vi "Compile Analog Replay Channels.vi"(5 "DAC bipolar range":dbl, 7 "Custom device ref":T1 format="%.0x", 8 "error in (no error)":errorcluster, 10 "1.0.0 Analog Replay in":T2, 11 "Item Ref in":T1 format="%.0x") -> (0 "error out":errorcluster, 2 "1.0.0 Analog Replay out":T2)   [LabVIEW 2013, in "Engine Simulation Toolkit System Explorer.lvlib"]
uses:
  Engine Simulation Toolkit System Explorer.lvlib
  Shared/1.0 Analog Replay Engine Data.ctl
  Shared/1.0 Analog Replay FIFO Idxs.ctl
  <vilib>/NI Veristand/Custom Device API/Custom Device Item Ref.ctl
  Shared/Constants and GUIDs.vi
  Shared/Properties.vi
  <vilib>/NI Veristand/Custom Device API/Get Item Property (Boolean).vi
  Shared/Engine Simulation Toolkit Shared.lvlib
  <vilib>/NI Veristand/Custom Device API/Custom Device API.lvlib
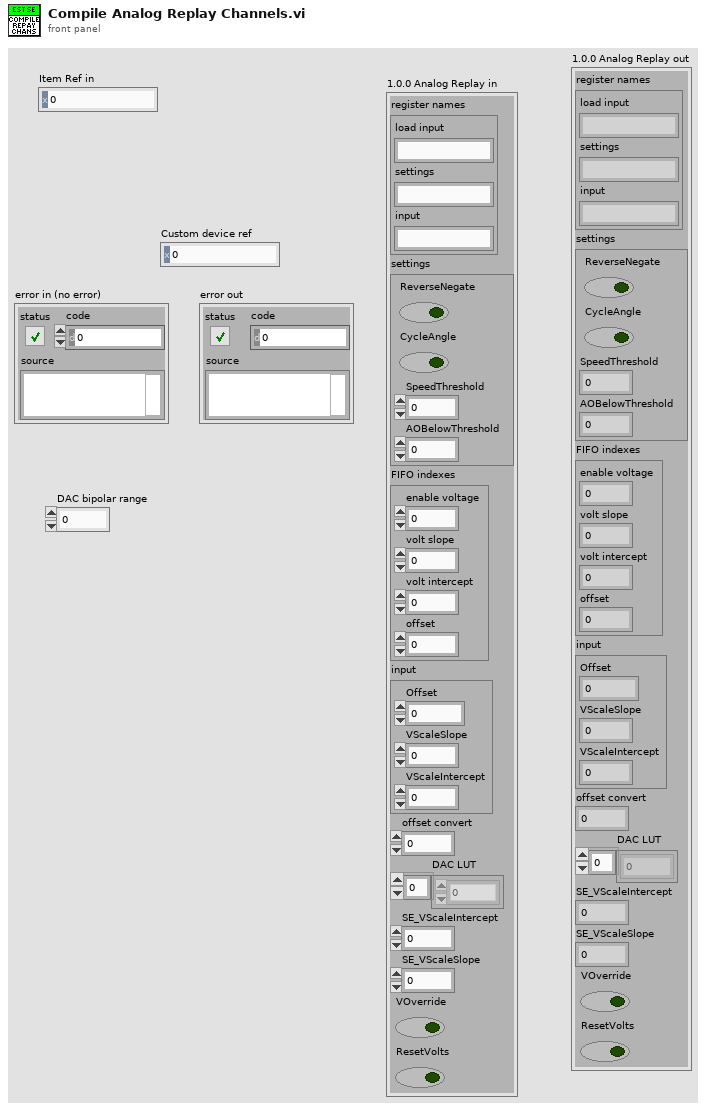
[diagram p1: front panel]
types:
  T1 = typedef "Custom Device API.lvlib/Custom Device Item Ref.ctl" = u64
  T2 = typedef "Engine Simulation Toolkit Shared.lvlib/1.0 Analog Replay Engine Data.ctl" = cluster{"register names":cluster{"load input":string, "settings":string, "input":string}, "settings":cluster{"ReverseNegate":bool, "CycleAngle":bool, "SpeedThreshold":fxp<+/-,23,2>, "AOBelowThreshold":i16}, "FIFO indexes":T3, "input":cluster{"Offset":i16, "VScaleSlope":fxp<+,18,6>, "VScaleIntercept":fxp<+/-,18,3>}, "offset convert":dbl, "DAC LUT":i16[], "SE_VScaleIntercept":fxp<+/-,18,3>, "SE_VScaleSlope":fxp<+,18,6>, "VOverride":bool, "ResetVolts":bool}
  T3 = typedef "Engine Simulation Toolkit Shared.lvlib/1.0 Analog Replay FIFO Idxs.ctl" = cluster{"enable voltage":i32, "volt slope":i32, "volt intercept":i32, "offset":i32}
  T4 = typedef "Engine Simulation Toolkit Shared.lvlib/Channel.ctl" = cluster{"Name":string, "Units":string, "Default":dbl, "Description":string}
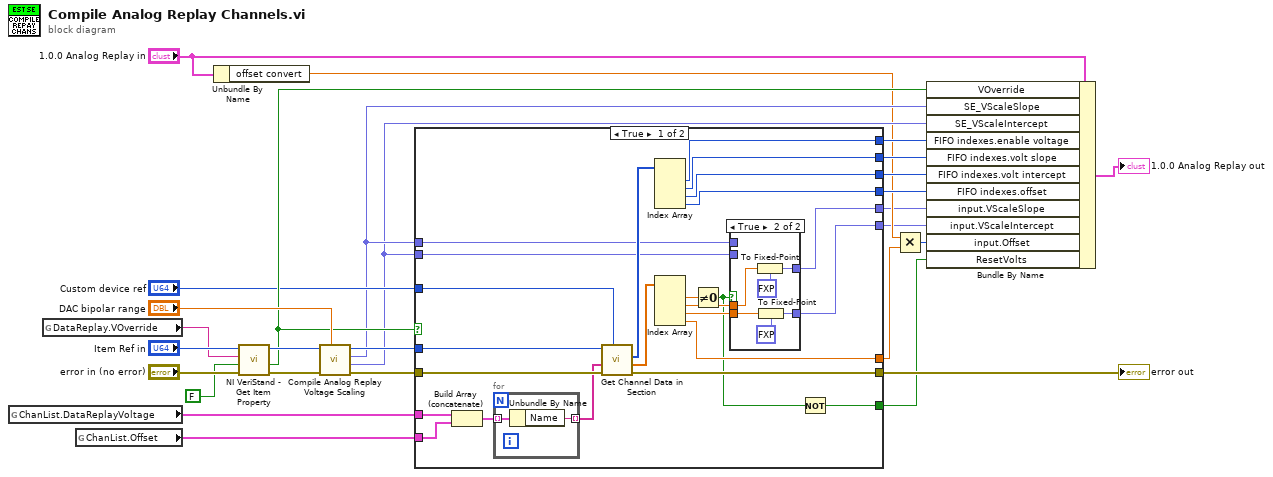
[diagram p0: block diagram]
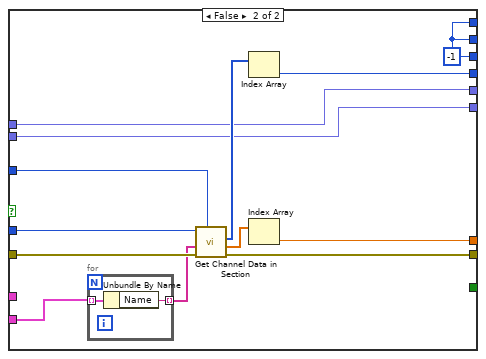
[diagram p3: hidden frame]
diagram:
  n1 = global read "Constants and GUIDs.vi" "ChanList.DataReplayVoltage"() -> (w20:T4[])
  n2 = global read "Properties.vi" "DataReplay.VOverride"() -> (w26:string)
  n3 = global read "Constants and GUIDs.vi" "ChanList.Offset"() -> (w19:T4[])
  n4 = Unbundle By Name("1.0.0 Analog Replay in") -> ("offset convert"=w5:dbl)
  n5 = call-poly <vilib>:"NI VeriStand - Get Item Property.vi"("error in (no error)"="error in (no error)", "Default Value"=FALSE, "Property Name"=w26, "Item Ref in"="Item Ref in") -> ("error out"=w23:errorcluster, "Value"=w21:bool, "Item Ref out"=w24:T1)  [unwired: 4 in, 1 out]
  n6 = call "Compile Analog Replay Voltage Scaling.vi"("DAC bipolar range"="DAC bipolar range", "error in (no error)"=w23, "Item Ref in"=w24) -> ("error out"=w17:errorcluster, "intercept (b)"=w8:fxp<+/-,18,3>, "slope (m)"=w9:fxp<+,18,6>, "Item Ref out"=w15:T1)  [unwired: 5 in]
  n7 = case shown="True" w21 {
    tunnel: w20 -> [w48 _]
    tunnel: w19 -> [w47 w68]
    tunnel: [w51 w74] -> w18
    tunnel: w17 -> [w52 w75]
    tunnel: w15 -> [w50 w73]
    tunnel: "Custom device ref" -> [w49 w72]
    tunnel: [w43 w63] -> w13
    tunnel: [w42 w63] -> w12
    tunnel: [w41 w63] -> w11
    tunnel: [w40 w66] -> w10
    tunnel: w9 -> [w32 w65]
    tunnel: w8 -> [w31 w64]
    tunnel: [w37 w67] -> w4
    tunnel: [w34 w64] -> w3
    tunnel: [w33 w65] -> w2
    tunnel: [w29 _] -> w1
    frame True {
      n8 = Build Array (concatenate)(w48, w47) -> (w46:T4[])
      n9 = for {
        tunnel: [w62] -> w45 mode=indexing
        tunnel: w46 -> [w61] mode=indexing
        n10 = Unbundle By Name(w61) -> ("Name"=w62:string)
      }
      n11 = call "Get Channel Data in Section.vi"("Custom device ref"=w49, "error in (no error)"=w52, "Channels"=w45, "Item Ref in"=w50) -> ("error out"=w51:errorcluster, "default values"=w39:dbl[], "FIFO indexes"=w44:i32[])  [unwired: 3 in, 2 out]
      n12 = Index Array(array=w44) -> (element #1=w43:i32, element #2=w42:i32, element #3=w41:i32, element #4=w40:i32)  [unwired: 4 in]
      n13 = Index Array(array=w39) -> (element #1=w38:dbl, element #2=w36:dbl, element #3=w35:dbl, element #4=w37:dbl)  [unwired: 4 in]
      n14 = Not Equal To 0?(x=w38) -> (x != 0?=w30:bool)
      n15 = case shown="True" w30 {
        tunnel: [w54 w58] -> w33
        tunnel: [w53 w57] -> w34
        tunnel: w36 -> [_ w56]
        tunnel: w35 -> [_ w55]
        tunnel: w32 -> [w54 _]
        tunnel: w31 -> [w53 _]
        frame False {
        }
        frame True {
          n16 = To Fixed-Point(fixed-point type=fxp<+,18,6> 0.0, number=w56) -> (fixed-point=w58:fxp<+,18,6>)
          n17 = To Fixed-Point(fixed-point type=fxp<+/-,18,3> 0.0, number=w55) -> (fixed-point=w57:fxp<+/-,18,3>)
        }
      }
      n18 = Not(x=w30) -> (.not. x?=w29:bool)
    }
    frame False {
      w63 = -1 ("Channel FIFO Buffer Index")
      n19 = for {
        tunnel: [w77] -> w71 mode=indexing
        tunnel: w68 -> [w76] mode=indexing
        n20 = Unbundle By Name(w76) -> ("Name"=w77:string)
      }
      n21 = call "Get Channel Data in Section.vi"("Custom device ref"=w72, "error in (no error)"=w75, "Channels"=w71, "Item Ref in"=w73) -> ("error out"=w74:errorcluster, "default values"=w69:dbl[], "FIFO indexes"=w70:i32[])  [unwired: 3 in, 2 out]
      n22 = Index Array(array=w70) -> (element=w66:i32)  [unwired: 1 in]
      n23 = Index Array(array=w69) -> (element=w67:dbl)  [unwired: 1 in]
    }
  }
  "error out" <- w18
  n24 = Multiply(x=w5, y=w4) -> (x*y=w6:i16)
  n25 = Bundle By Name(cluster="1.0.0 Analog Replay in", "VOverride"=w21, "SE_VScaleSlope"=w9, "SE_VScaleIntercept"=w8, "FIFO indexes.enable voltage"=w13, "FIFO indexes.volt slope"=w12, "FIFO indexes.volt intercept"=w11, "FIFO indexes.offset"=w10, "input.VScaleSlope"=w2, "input.VScaleIntercept"=w3, "input.Offset"=w6, "ResetVolts"=w1) -> (→"1.0.0 Analog Replay out":T2)
